vi "Acquire Result.vi"(8 "error in (no error)":errorcluster, 11 "Mag Lab Measurement in":refnum<class "Mag Lab Measurement.lvclass">) -> (0 "error out":errorcluster, 3 "Mag Lab Measurement out":refnum<class "Mag Lab Measurement.lvclass">)   [LabVIEW 2015, in "Mag Lab Measurement.lvclass"]
uses:
  Mag Lab Measurement.lvclass
  Mag Lab Measurement.lvclass/Mag Lab Measurement.ctl
  Mag Lab Error Handler/Mag Lab Error Handler.lvclass
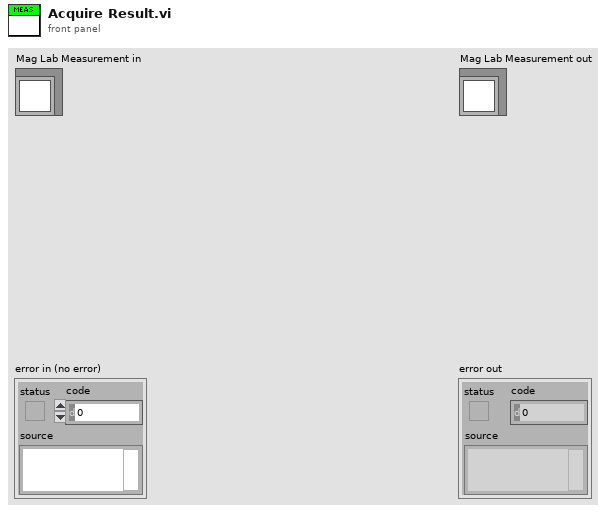
[diagram p1: front panel]
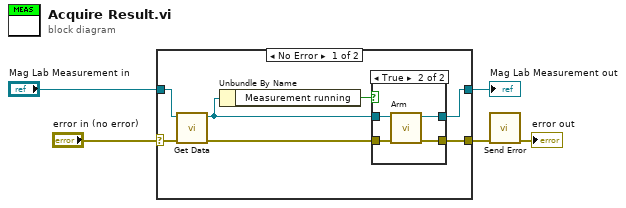
[diagram p0: block diagram]
diagram:
  n1 = case shown="No Error" "error in (no error)" {
    selector: "error in (no error)" -> [w9 w20]
    tunnel: [w7 w20] -> w2
    tunnel: [w6 w19] -> w3
    tunnel: "Mag Lab Measurement in" -> [w12 w19]
    frame No Error {
      n2 = call-dynamic "Get Data.vi"("error in (no error)"=w9, "Mag Lab Measurement in"=w12) -> ("error out"=w8:errorcluster, "Mag Lab Measurement out"=w10:refnum<class "Mag Lab Measurement.lvclass">)  [unwired: 8 in]
      n3 = Unbundle By Name(w10) -> ("Measurement running"=w11:bool)
      n4 = case shown="True" w11 {
        tunnel: w10 -> [w13 w18]
        tunnel: w8 -> [w14 w17]
        tunnel: [w14 w16] -> w7
        tunnel: [w13 w15] -> w6
        frame False {
        }
        frame True {
          n5 = call-dynamic "Arm.vi"("error in (no error)"=w17, "Mag Lab Measurement in"=w18) -> ("error out"=w16:errorcluster, "Mag Lab Measurement out"=w15:refnum<class "Mag Lab Measurement.lvclass">)  [unwired: 8 in]
        }
      }
    }
    frame Error {
    }
  }
  "Mag Lab Measurement out" <- w3
  n6 = call "Send Error.vi"("error in (no error)"=w2) -> ("error out"=→"error out":errorcluster)  [unwired: 9 in, 1 out]
